vi "Lift Wrapper.vi"(8 "Fast And Furious":bool, 10 "Lift down":bool, 11 "Lift up":bool) -> ()   [LabVIEW 2014]
uses:
  Precreated VIs/Robot Global Data.vi
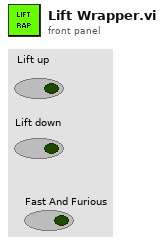
[diagram p1: front panel]
types:
  T1 = cluster{"Distance":dbl, "Rate":dbl, "Direction":bool, "Stopped":bool}
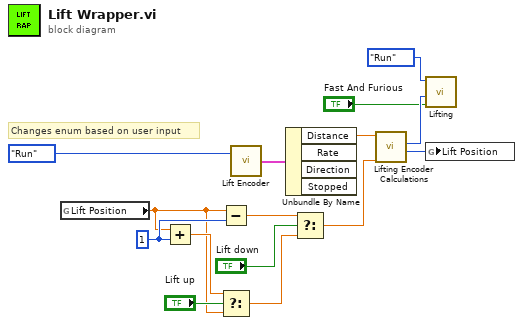
[diagram p0: block diagram]
diagram:
  w6 = 1
  # "Changes enum based on user input"
  n1 = global read "Robot Global Data.vi" "Lift Position"() -> (w5:dbl)
  n2 = Add(x=w5, y=w6) -> (x+y=w9:dbl)
  n3 = Subtract(x=w5, y=w6) -> (x-y=w8:dbl)
  n4 = Select(t=w9, s="Lift up", f=w5) -> (s? t:f=w7:dbl)
  n5 = call "Lift Encoder.vi"("Mode"=enum8{"Start", "Run", "Finish"}."Run") -> ("Lift Encoder"=w14:T1)  [unwired: 1 in]
  n6 = Unbundle By Name(w14) -> ("Distance"=w13:dbl)  [unwired: 3 out]
  n7 = Select(t=w8, s="Lift down", f=w7) -> (s? t:f=w10:dbl)
  n8 = call "Lifting Encoder Calculations.vi"("Desired Position"=w10, "Height (from encoder)"=w13) -> ("Current position"=w4:i32, "Direction"=w2:enum16{"stop", "up", "down"})  [unwired: 7 in]
  n9 = call "Lifting.vi"("Fast And Furious"="Fast And Furious", "Direction"=w2, "Mode"=enum8{"Start", "Run", "Finish"}."Run") -> ()  [unwired: 4 in]
  n10 = global write "Robot Global Data.vi" "Lift Position"(w4) -> ()
